vi "Project.vi"() -> ()   [LabVIEW 2020]
uses:
  <vilib>/MakerHub/LINX/Public/Peripherals/PWM/PWM Set Duty Cycle 1 Chan.vi
  <vilib>/MakerHub/LINX/Public/Peripherals/Analog/Analog Read 1 Chan.vi
  <vilib>/MakerHub/LINX/Public/Peripherals/Analog/Analog Read N Chans.vi
  <vilib>/MakerHub/LINX/Private/Local IO/LinxAnalogRead.vi
  <vilib>/MakerHub/LINX/Public/Utilities/Check Channel.vi
  <vilib>/MakerHub/LINX/Public/Utilities/Open Serial.vi
  <userlib>/_OpenG.lib/comparison/comparison.llb/U8 Changed__ogtk.vi
  <userlib>/_OpenG.lib/comparison/comparison.llb/Boolean Changed__ogtk.vi
  <vilib>/MakerHub/LINX/Public/Peripherals/PWM/PWM Set Duty Cycle N Chans.vi
  <vilib>/MakerHub/LINX/Private/Utilties/Generate Error.vi
  <vilib>/MakerHub/LINX/LMH-LINX.lvlib
panel:
  in  "Water Sensor Channel":u8
  in  "Fan Channel":u8=3
  in  "LED Channel":u8=5
  in  "Photodioe hannel":u8
  in  "Serial Port":refnum<visa-resource-name>="N/A"
  in  "stop":bool
  in  "Max Temperature (C)":dbl=30.0
  out "System Humidity":dbl[](graph)
  out "System Temperature":dbl[](graph)
  out "Light Status":bool
  in  "Light End":timestamp=timestamp(7200 s since 1904-01-01) format="%<%I:%M %p>T"
  in  "Light Start Stamp":timestamp=timestamp(-43200 s since 1904-01-01) format="%<%I:%M %p>T"
  in  "Desired Water Level":dbl(slide)=8.061224489795919 scale=0.0..10.0
  in  "Max Humidity (%)":dbl=40.0
  out "Environment Temperature (C)":u8=21
  out "Environment Humidity (%)":u8=35
  out "System Humidity (%)":u8
  out "System Temperature (C)":u8
  out "Water Level":dbl(slide) scale=0.0..10.0
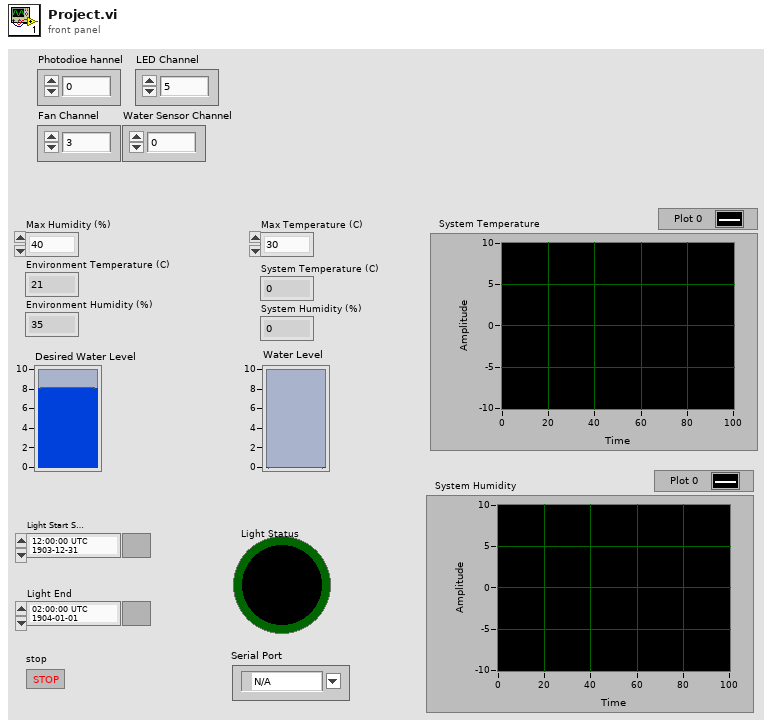
[diagram p1: front panel]
types:
  T1 = typedef "LMH-LINX.lvlib/LINX Ref.ctl" = cluster{"IO":T2, "Interface":T3, "LINX Device Config":T4}
  T2 = typedef "LMH-LINX.lvlib/Platform.ctl" = enum16{"Remote", "Local"}
  T3 = typedef "LMH-LINX.lvlib/Interface.ctl" = enum16{"Serial", "TCP"}
  T4 = typedef "LMH-LINX.lvlib/Device.lvlib/LINX Device Config.ctl" = cluster{"Interface":T3, "COM Port":refnum<visa-resource-name>, "TCP Configuration":T5, "Device Family":u8, "Device ID":u8, "Device Name":string, "TCP Ref":refnum<k5>, "Channels":T6}
  T5 = typedef "LMH-LINX.lvlib/Device.lvlib/TCP Config.ctl" = cluster{"IP Address":string, "Port":u16}
  T6 = typedef "LMH-LINX.lvlib/Channels.ctl" = cluster{"DI":u8[], "DO":u8[], "AI":u8[], "AO":u8[], "PWM":u8[], "QE":u8[], "UART":u8[], "I2C 2":u8[], "SPI":u8[], "CAN":u8[], "Servo":u8[], "AI Ref (V)":dbl, "AI Resolution (Bits)":u8, "AO Ref (V)":dbl, "AO Resolution (Bits)":u8}
  T7 = cluster{"Water Sensor Channel":u8, "LED Channel":u8, "Photodioe hannel":u8, "Fan Channel":u8}
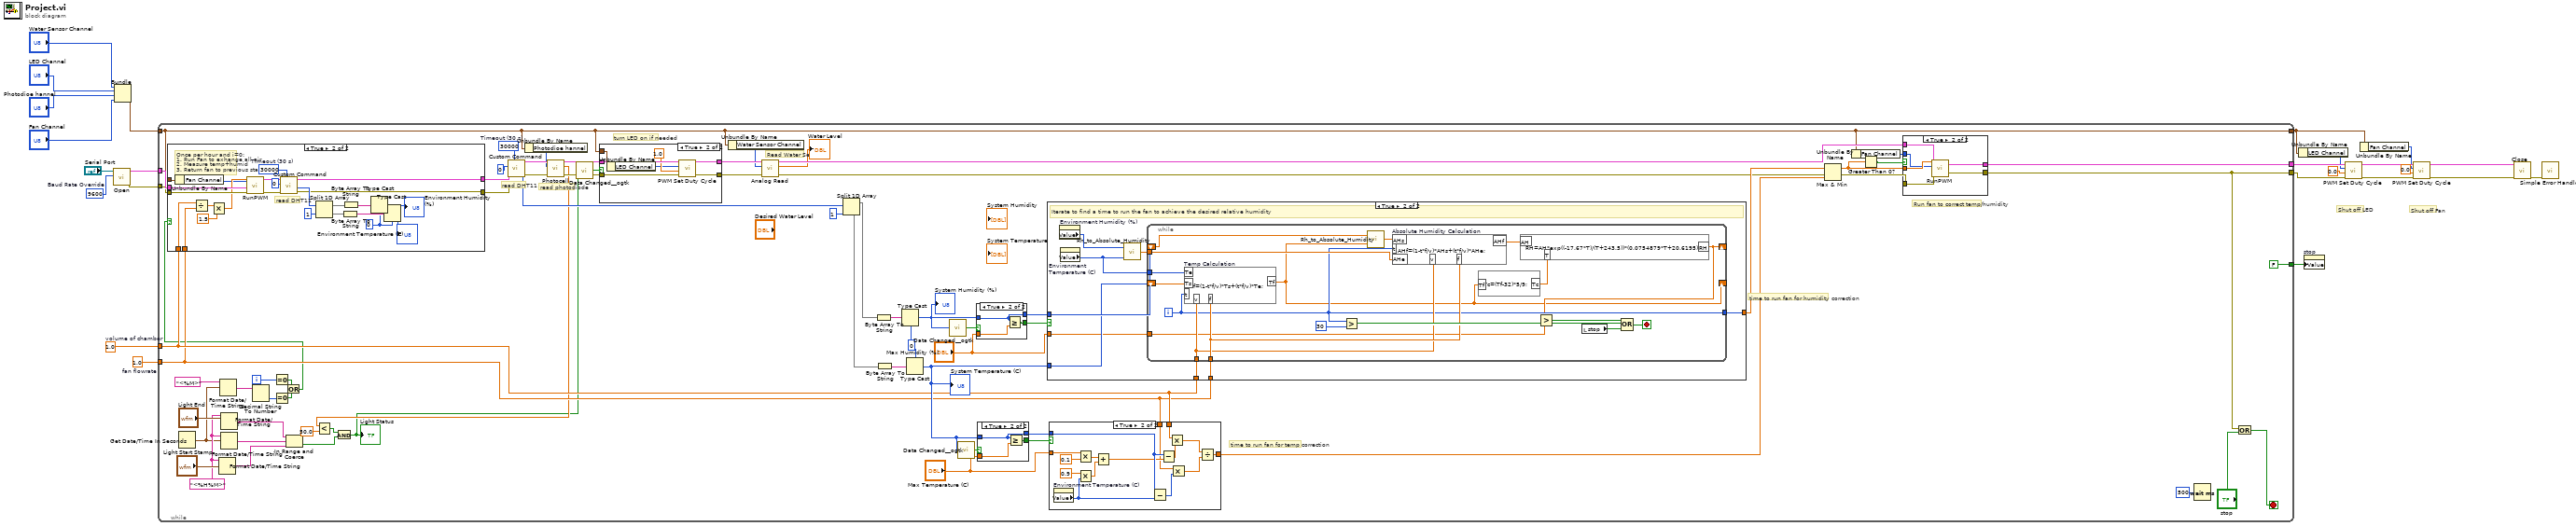
[diagram p0: block diagram]
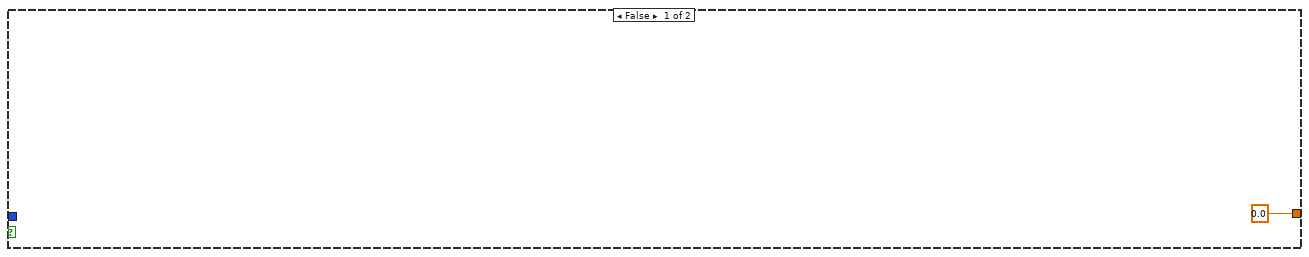
[diagram p4: hidden frame]
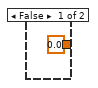
[diagram p5: hidden frame]
diagram:
  w19 = 1.0  # fan flowrate
  w20 = 1.0  # volume of chamber
  w23 = u32 9600  # Baud Rate Override
  # "Shut off Fan"
  # "Shut off LED"
  n1 = call-poly <vilib>:"Open.vi"("Baud Rate Override"=w23, "Serial Port"="Serial Port") -> ("Error Out"=w21:errorcluster, "LINX Resource"=w22:T1)  [unwired: 7 in, 1 out]
  n2 = Bundle("Water Sensor Channel"="Water Sensor Channel", "LED Channel"="LED Channel", "Photodioe hannel"="Photodioe hannel", "Fan Channel"="Fan Channel") -> (w5:T7)  [unwired: 1 in]
  n3 = while {
    tunnel: w22 -> [w61]
    tunnel: w21 -> [w60]
    tunnel: [w44] -> w17
    tunnel: w20 -> [w63]
    tunnel: w19 -> [w62]
    tunnel: [w37] -> w16
    tunnel: w5 -> [w29]
    tunnel: [w29] -> w2
    tunnel: [FALSE] -> w1
    i -> [w43]
    stop <- w39 stop-if-true
    w27 = u8 0
    w65 = 30000  # Timeout (30 s)
    w87 = "<%H%M>"
    # "Read Water Sensor"
    # "Run fan to correct temp/humidity"
    # "turn LED on if needed"
    # "read photodiode"
    # "read DHT11"
    # "time to run fan for humidity correction"
    # "time to run fan for temp correction"
    n4 = Get Date/Time In Seconds() -> (seconds since 1Jan1904=w85:timestamp)
    n5 = Format Date/Time String(time format string (%c)=w87, seconds (now)="Light Start Stamp") -> (date/time string=w90:string)  [unwired: 1 in]
    n6 = Format Date/Time String(time format string (%c)="<%M>", seconds (now)=w85) -> (date/time string=w84:string)  [unwired: 1 in]
    n7 = Format Date/Time String(time format string (%c)=w87, seconds (now)="Light End") -> (date/time string=w91:string)  [unwired: 1 in]
    n8 = Format Date/Time String(time format string (%c)=w87, seconds (now)=w85) -> (date/time string=w89:string)  [unwired: 1 in]
    n9 = Decimal String To Number(string=w84) -> (number=w83:i32)  [unwired: 2 in, 1 out]
    n10 = Equal To 0?(x=w43) -> (x = 0?=w42:bool)
    n11 = Equal To 0?(x=w83) -> (x = 0?=w41:bool)
    n12 = Or(x=w42, y=w41) -> (x .or. y?=w40:bool)
    n13 = case shown="True" w40 {
      tunnel: w60 -> [w164 w176]
      tunnel: w61 -> [w165 w177]
      tunnel: [w165 w179] -> w59
      tunnel: [w164 w178] -> w58
      tunnel: w63 -> [_ w172]
      tunnel: w62 -> [_ w171]
      tunnel: w29 -> [_ w167]
      frame False {
      }
      frame True {
        w166 = u8 0
        w188 = 30000  # Timeout (30 s)
        # "read DHT11"
        # "Once per hour and i=0:\n1. Run Fan to exhange all air\n2. Measure temp+humid\n3. Return fan to previous state"
        n14 = Unbundle By Name(w167) -> ("Fan Channel"=w168:u8)
        n15 = Divide(x=w172, y=w171) -> (x/y=w173:dbl)
        n16 = Multiply(x=w173, y=1.5) -> (x*y=w174:dbl)
        n17 = call "RunPWM.vi"("Error In"=w176, "LINX In"=w177, "PWM Channel"=w168, "Seconds To Run"=w174) -> ("Error Out"=w170:errorcluster, "LINX Out"=w169:T1)
        n18 = call <vilib>:"Custom Command.vi"("Timeout (100 ms)"=w188, "Error In"=w170, "Custom Command Number"=u16 0, "LINX Resource"=w169) -> ("Error Out"=w178:errorcluster, "Response"=w187:u8[], "LINX Resource"=w179:T1)  [unwired: 4 in, 1 out]
        n19 = Split 1D Array(array=w187, index=1) -> (first subarray=w183:u8[], second subarray=w182:u8[])
        n20 = Byte Array To String(unsigned byte array=w182) -> (string=w184:string)
        n21 = Byte Array To String(unsigned byte array=w183) -> (string=w185:string)
        n22 = Type Cast(type=w166, x=w185) -> (*(type *) &x=→"Environment Humidity (%)":u8)
        n23 = Type Cast(type=w166, x=w184) -> (*(type *) &x=→"Environment Temperature (C)":u8)
      }
    }
    n24 = In Range and Coerce(upper limit=w91, x=w89, lower limit=w90) -> (In Range?=w52:bool)  [unwired: 1 out]
    n25 = call <vilib>:"Custom Command.vi"("Timeout (100 ms)"=w65, "Error In"=w58, "Custom Command Number"=u16 0, "LINX Resource"=w59) -> ("Error Out"=w57:errorcluster, "Response"=w71:u8[], "LINX Resource"=w56:T1)  [unwired: 4 in, 1 out]
    n26 = Unbundle By Name(w29) -> ("Photodioe hannel"=w28:u8)
    n27 = call <vilib>:"Photocell.vi"("Error In"=w57, "AI Channel"=w28, "LINX Resource"=w56) -> ("Error Out"=w54:errorcluster, "Value (0-100)"=w53:dbl, "LINX Resource"=w55:T1)  [unwired: 6 in]
    n28 = Less?(x=w53, y=50.0) -> (x < y?=w51:bool)
    n29 = And(x=w51, y=w52) -> (x .and. y?=w49:bool)
    "Light Status" <- w49
    n30 = call-poly <userlib>:"Data Changed__ogtk.vi"("Boolean"=w49) -> ("Changed"=w50:bool)
    n31 = case shown="True" w50 {
      tunnel: w55 -> [w102 w109]
      tunnel: w54 -> [w101 w108]
      tunnel: [w102 w107] -> w35
      tunnel: [w101 w106] -> w33
      tunnel: w29 -> [_ w104]
      frame False {
      }
      frame True {
        n32 = Unbundle By Name(w104) -> ("LED Channel"=w103:u8)
        n33 = call-poly <vilib>:"PWM Set Duty Cycle.vi"("Error In"=w108, "Duty Cycle (0-1)"=1.0, "PWM Channel"=w103, "LINX Resource"=w109) -> ("Error Out"=w106:errorcluster, "LINX Resource"=w107:T1)  [unwired: 6 in]
      }
    }
    n34 = Unbundle By Name(w29) -> ("Water Sensor Channel"=w30:u8)
    n35 = call-poly <vilib>:"Analog Read.vi"("Error In"=w33, "Analog Channel"=w30, "LINX Resource"=w35) -> ("Error Out"=w34:errorcluster, "Voltage"=→"Water Level":dbl, "LINX Resource"=w36:T1)  [unwired: 5 in, 1 out]
    n36 = Split 1D Array(array=w71, index=1) -> (first subarray=w69:u8[], second subarray=w68:u8[])
    n37 = Byte Array To String(unsigned byte array=w69) -> (string=w67:string)
    n38 = Byte Array To String(unsigned byte array=w68) -> (string=w66:string)
    n39 = Type Cast(type=w27, x=w67) -> (*(type *) &x=w25:u8)
    "System Humidity (%)" <- w25
    n40 = Type Cast(type=w27, x=w66) -> (*(type *) &x=w64:u8)
    "System Temperature (C)" <- w64
    n41 = call-poly <userlib>:"Data Changed__ogtk.vi"("U8"=w25) -> ("Changed"=w81:bool)
    n42 = call-poly <userlib>:"Data Changed__ogtk.vi"("U8"=w64) -> ("Changed"=w80:bool)
    n43 = case shown="True" w81 {
      selector: w81 -> [w160 _]
      tunnel: w25 -> [w159 w162]
      tunnel: [w160 w163] -> w75
      tunnel: [w159 w162] -> w73
      tunnel: "Max Humidity (%)" -> [_ w161]
      frame False {
      }
      frame True {
        n44 = Greater Or Equal?(x=w162, y=w161) -> (x >= y?=w163:bool)
      }
    }
    n45 = case shown="True" w80 {
      selector: w80 -> [w155 _]
      tunnel: w64 -> [w154 w157]
      tunnel: [w155 w158] -> w79
      tunnel: [w154 w157] -> w78
      tunnel: "Max Temperature (C)" -> [_ w156]
      frame False {
      }
      frame True {
        n46 = Greater Or Equal?(x=w157, y=w156) -> (x >= y?=w158:bool)
      }
    }
    n47 = case shown="True" w75 {
      tunnel: w73 -> [_ w119]
      tunnel: [0.0 w112] -> w48
      tunnel: "Max Humidity (%)" -> [_ w111]
      tunnel: w64 -> [_ w118]
      tunnel: w63 -> [_ w116]
      tunnel: w62 -> [_ w115]
      frame False {
      }
      frame True {
        # "Iterate to find a time to run the fan to achieve the desired relative humidity"
        n48 = property on="Environment Humidity (%)" class="DigNum (strict)"() -> ("Value"=w114:u8)  [unwired: 2 in, 2 out]
        n49 = property on="Environment Temperature (C)" class="DigNum (strict)"() -> ("Value"=w117:u8)  [unwired: 2 in, 2 out]
        n50 = call "Rh_to_Absolute_Humidity.vi"("Temperature (F)"=w117, "Relative Humidity"=w114) -> ("Absolute Humidity"=w113:dbl)
        n51 = while {
          tunnel: w117 -> [w132]
          tunnel: w116 -> [w129]
          tunnel: w115 -> [w130]
          shift-right: [w122] -> _
          shift-left: w118 -> [w137]
          tunnel: w113 -> [w128]
          shift-right: [w125] -> _
          shift-left: w119 -> [w133]
          tunnel: [w127] -> w112
          tunnel: w111 -> [w124]
          i -> [w127]
          stop <- w136 stop-if-true
          n52 = formula code="Tf=(1-t*f/v)*Ts+(t*f/v)*Te;" "Temp Calculation"("Te"=w132, "Ts"=w137, "t"=w127, "v"=w129, "f"=w130) -> ("Tf"=w122:dbl)
          n53 = Greater?(x=w127, y=30) -> (0:w135:bool)
          n54 = call "Rh_to_Absolute_Humidity.vi"("Temperature (F)"=w122, "Relative Humidity"=w133) -> ("Absolute Humidity"=w131:dbl)
          n55 = formula code="AHf=(1-t*f/v)*AHs+(t*f/v)*AHe;" "Absolute Humidity Calculation"("AHs"=w131, "AHe"=w128, "v"=w129, "f"=w130, "t"=w127) -> ("AHf"=w126:dbl)
          n56 = formula code="Tc=(Tf-32)*5/9;"("Tf"=w122) -> ("Tc"=w121:dbl)
          n57 = formula code="RH=AH*exp((-17.67*T)/(T+243.5))*(0.0754879*T+20.6195);"("AH"=w126, "T"=w121) -> ("RH"=w125:dbl)
          n58 = Greater?(x=w125, y=w124) -> (0:w123:bool)
          n59 = local read "stop"() -> (w120:bool)
          n60 = Compound Arithmetic op=OR(w123, w135, w120) -> (w136:bool)
        }
      }
    }
    n61 = case shown="True" w79 {
      tunnel: w78 -> [_ w148]
      tunnel: [0.0 w153] -> w47
      tunnel: "Max Temperature (C)" -> [_ w147]
      tunnel: w62 -> [_ w140]
      tunnel: w63 -> [_ w139]
      frame False {
      }
      frame True {
        n62 = property on="Environment Temperature (C)" class="DigNum (strict)"() -> ("Value"=w146:u8)  [unwired: 2 in, 2 out]
        n63 = Multiply(x=w147, y=0.1) -> (x*y=w143:dbl)
        n64 = Multiply(x=0.9, y=w146) -> (x*y=w142:dbl)
        n65 = Add(x=w143, y=w142) -> (x+y=w141:dbl)
        n66 = Subtract(x=w148, y=w146) -> (x-y=w150:u8)
        n67 = Subtract(x=w148, y=w141) -> (x-y=w149:dbl)
        n68 = Multiply(x=w139, y=w149) -> (x*y=w151:dbl)
        n69 = Multiply(x=w140, y=w150) -> (x*y=w152:dbl)
        n70 = Divide(x=w151, y=w152) -> (x/y=w153:dbl)
      }
    }
    n71 = Max & Min(x=w48, y=w47) -> (max(x,y)=w45:dbl)  [unwired: 1 out]
    n72 = Unbundle By Name(w29) -> ("Fan Channel"=w31:u8)
    n73 = Greater Than 0?(x=w45) -> (x > 0?=w46:bool)
    n74 = case shown="True" w46 {
      tunnel: w45 -> [_ w96]
      tunnel: [w94 w100] -> w44
      tunnel: [w93 w99] -> w37
      tunnel: w36 -> [w94 w98]
      tunnel: w34 -> [w93 w97]
      tunnel: w31 -> [_ w95]
      frame False {
      }
      frame True {
        n75 = call "RunPWM.vi"("Error In"=w97, "LINX In"=w98, "PWM Channel"=w95, "Seconds To Run"=w96) -> ("Error Out"=w99:errorcluster, "LINX Out"=w100:T1)
      }
    }
    n76 = Wait (ms)(milliseconds to wait=u32 500) -> ()  [unwired: 1 out]
    n77 = Compound Arithmetic op=OR(w37, "stop") -> (w39:bool)
  }
  n78 = Unbundle By Name(w2) -> ("LED Channel"=w3:u8)
  n79 = property on="stop" class="Bool (strict)"("Value"=w1) -> ()  [unwired: 2 in, 2 out]
  n80 = call-poly <vilib>:"PWM Set Duty Cycle.vi"("Error In"=w16, "Duty Cycle (0-1)"=0.0, "PWM Channel"=w3, "LINX Resource"=w17) -> ("Error Out"=w14:errorcluster, "LINX Resource"=w15:T1)  [unwired: 6 in]
  n81 = Unbundle By Name(w2) -> ("Fan Channel"=w4:u8)
  n82 = call-poly <vilib>:"PWM Set Duty Cycle.vi"("Error In"=w14, "Duty Cycle (0-1)"=0.0, "PWM Channel"=w4, "LINX Resource"=w15) -> ("Error Out"=w12:errorcluster, "LINX Resource"=w10:T1)  [unwired: 6 in]
  n83 = call <vilib>:"Close.vi"("Error In"=w12, "LINX Resource"=w10) -> ("Error Out"=w11:errorcluster)  [unwired: 9 in]
  n84 = call <vilib>:"Simple Error Handler.vi"("error in (no error)"=w11) -> ()  [unwired: 4 in, 5 out]
